vi "NI VeriStand - Search for Item.vi"   [LabVIEW 2020, in "Custom Device Utility Library.lvlib"]
doc: "Searches a custom device section for the item(s) you specify. You can search for one or multiple items by name, GUID, or property name and value. You must manually select the polymorphic instance to use."
uses:
  <vilib>/NI VeriStand/Custom Device Tools/Custom Device Utility Library/Custom Device Utility Library.lvlib
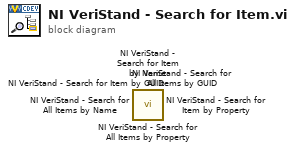
[diagram p0: block diagram]
diagram:
  n1 = call <vilib>:"NI VeriStand - Search for All Items by Property.vi"() -> ()  [unwired: 8 in, 4 out]
  n2 = call <vilib>:"NI VeriStand - Search for All Items by GUID.vi"() -> ()  [unwired: 8 in, 4 out]
  n3 = call <vilib>:"NI VeriStand - Search for All Items by Name.vi"() -> ()  [unwired: 8 in, 4 out]
  n4 = call <vilib>:"NI VeriStand - Search for Item by Property.vi"() -> ()  [unwired: 8 in, 4 out]
  n5 = call <vilib>:"NI VeriStand - Search for Item by GUID.vi"() -> ()  [unwired: 8 in, 4 out]
  n6 = call <vilib>:"NI VeriStand - Search for Item by Name.vi"() -> ()  [unwired: 8 in, 4 out]
